vi "Shooter_Begin.vi"   [LabVIEW 2020]
uses:
  Shooter_Control_States.ctl
  Subsystems/Cowl/Cowl_States.ctl
  Subsystems/Cowl/Cowl_Cluster.ctl
  Subsystems/Flywheel/Flywheel_States.ctl
  Subsystems/Flywheel/Flywheel_Cluster.ctl
  Subsystems/Turret/Turret_States.ctl
  Subsystems/Turret/Turret_Cluster.ctl
  Determiner_Begin_Cluster.ctl
  Shooter_Globals.vi
types:
  T1 = typedef "Determiner_Begin_Cluster.ctl" = cluster{"Turret_Cluster":T2, "Flywheel_Cluster":T4, "Shooter_Control_State":T6, "Cowl_Cluster":T7, "Shooting?":bool, "Upper_Goal?":bool, "Lower_Goal?":bool, "Shooting":bool}
  T2 = typedef "Turret_Cluster.ctl" = cluster{"Auto-Target?":bool, "Turret_Control_State":T3, "Turret_Spin_Speed":dbl, "Turret_Spin_Speed_Control?":bool, "Step":dbl, "Parameter_1":dbl, "Parameter_2":dbl, "Parameter_3":dbl, "Auto_Notifier":refnum<notifier>, "GoToZero?":bool}
  T3 = typedef "Turret_States.ctl" = enum16{"Manual_Percent_Voltage", "Manual_Speed_Control", "Auto-Target", "Command_TurnToPosition", "Command_Auto_Target", "GoToZero"}
  T4 = typedef "Flywheel_Cluster.ctl" = cluster{"Flywheel_Throttle":dbl, "Flywheel_Control_State":T5, "Auto_Speed":bool, "Flywheel_On":bool, "Parameter_1":dbl, "Parameter_2":dbl, "Auto_Notifier":refnum<notifier>, "Step":dbl}
  T5 = typedef "Flywheel_States.ctl" = enum16{"No-Op", "Percent_Voltage", "Speed_Control_Manual", "Speed_Control_Auto", "Command_SpinUp", "Command_SpinUpAuto"}
  T6 = typedef "Shooter_Control_States.ctl" = enum16{"No-Op", "Limelight_Shooting", "Low_Goal", "High_Goal", "Shoot_From_Pose"}
  T7 = typedef "Cowl_Cluster.ctl" = cluster{"Cowl_Control_State":T8, "Manual_Cowl_%Power":dbl}
  T8 = typedef "Cowl_States.ctl" = enum16{"Manual_%VBus", "GoToAngle"}
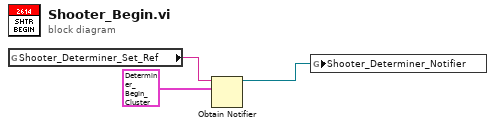
[diagram p0: block diagram]
diagram:
  n1 = global read "Shooter_Globals.vi" "Shooter_Determiner_Set_Ref"() -> (w2:string)
  n2 = Obtain Notifier(name (unnamed)=w2, notification data type=T1 {"Turret_Cluster"={"Auto-Target?"=FALSE, "Turret_Control_State"=enum."Manual_Percent_Voltage", "Turret_Spin_Speed"=0.0, "Turret_Spin_Speed_Control?"=FALSE, "Step"=0.0, "Parameter_1"=0.0, "Parameter_2"=0.0, "Parameter_3"=0.0, "Auto_Notifier"=refnum, "GoToZero?"=FALSE}, "Flywheel_Cluster"={"Flywheel_Throttle"=0.0, "Flywheel_Control_State"=enum."No-Op", "Auto_Speed"=FALSE, "Flywheel_On"=FALSE, "Parameter_1"=0.0, "Parameter_2"=0.0, "Auto_Notifier"=refnum, "Step"=0.0}, "Shooter_Control_State"=enum."No-Op", "Cowl_Cluster"={"Cowl_Control_State"=enum."Manual_%VBus", "Manual_Cowl_%Power"=0.0}, "Shooting?"=FALSE, "Upper_Goal?"=FALSE, "Lower_Goal?"=FALSE, "Shooting"=FALSE}) -> (notifier out=w3:refnum<notifier>)  [unwired: 2 in, 2 out]
  n3 = global write "Shooter_Globals.vi" "Shooter_Determiner_Notifier"(w3) -> ()
